vi "Add UIPs.vi"(8 "Error In":errorcluster, 9 "Enabled (True)":bool[](array[boolean]), 10 "UIPs":refnum<class "UIP Interface.lvclass">[](array[class]), 11 "UIM In":refnum<data-value>) -> (0 "Error Out":errorcluster, 3 "UIM Out":refnum<data-value>)   [LabVIEW 2020, in "UIM.lvlib" / "UIM.lvclass"]
doc: "Specify a list of UIPs to be loaded. They are enabled by default. The new UIPs are appended to the ones already loaded."
uses:
  UIM.lvclass
  UIP Interface/UIP Interface.lvclass
  UIM.lvclass/UIM.ctl
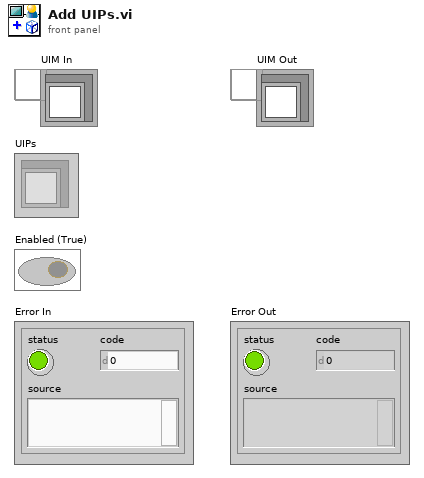
[diagram p1: front panel]
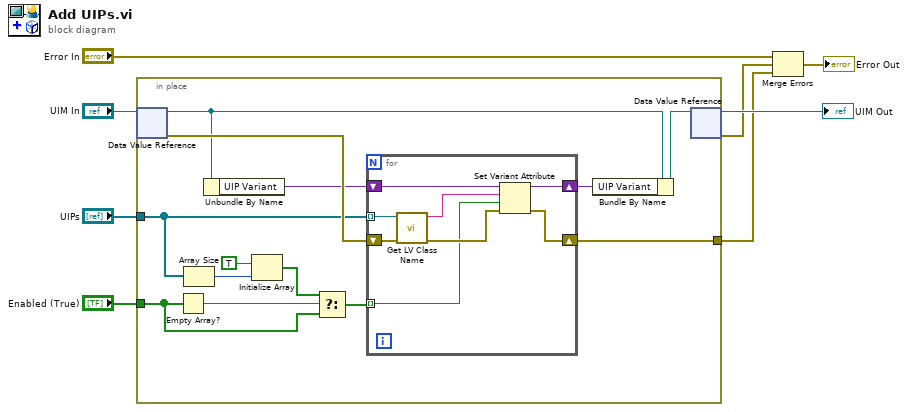
[diagram p0: block diagram]
diagram:
  n1 = in-place {
    in-place-border: [w20] -> w3
    in-place-border: "UIPs" -> [w14]
    in-place-border: "Enabled (True)" -> [w10]
    n2 = in-place-dvr #1("UIM In") -> (w18:refnum<class "UIM.lvclass">, w21:errorcluster)
    n3 = Empty Array?(array=w10) -> (empty?=w12:bool)
    n4 = Array Size(array=w14) -> (size(s)=w15:i32)
    n5 = Unbundle By Name(w18) -> ("UIP Variant"=w19:variant)
    n6 = Initialize Array(TRUE, w15) -> (w11:bool[])
    n7 = Select(t=w11, s=w12, f=w10) -> (s? t:f=w9:bool[])
    n8 = for {
      tunnel: w14 -> [w26] mode=indexing
      shift-right: [w29] -> w20
      shift-left: w21 -> [w23]
      shift-right: [w27] -> w16
      shift-left: w19 -> [w28]
      tunnel: w9 -> [w22] mode=indexing
      n9 = call <vilib>:"Get LV Class Name.vi"("error in (no error)"=w23, "object"=w26) -> ("error out"=w24:errorcluster, "class name"=w25:string)  [unwired: 8 in]
      n10 = Set Variant Attribute(Variant=w28, name=w25, value=w22, error in=w24) -> (Variant out=w27:variant, error out=w29:errorcluster)  [unwired: 1 out]
    }
    n11 = Bundle By Name(cluster=w18, "UIP Variant"=w16) -> (w17:refnum<class "UIM.lvclass">)
    n12 = in-place-dvr #1(w17) -> (→"UIM Out":refnum<data-value>, w2:errorcluster)
  }
  n13 = Merge Errors("Error In", w2, w3) -> (→"Error Out":errorcluster)
